vi "CuLab_FM_Demodulate.vi"(8 "error in (no error)":errorcluster, 11 "Signal In":refnum<class "T1D_CSG.lvclass">) -> (0 "error out":errorcluster, 3 "FM Demod Out":refnum<class "T1D_SGL.lvclass">)   [LabVIEW 2020]
uses:
  <vilib>/Ngene/CuLab - GPU Accelerated Toolkit/Toolkit/Low_Level/Tensor_Classes/T_Children/T1D/T1D_Children/T1D_CSG/T1D_CSG.lvclass
  C:/Program Files/National Instruments/LabVIEW 2020/vi.lib/Ngene/CuLab - GPU Accelerated Toolkit/Toolkit/Low_Level/Tensor_Classes/T_Children/T1D/T1D.lvclass
  <vilib>/Ngene/CuLab - GPU Accelerated Toolkit/Toolkit/Low_Level/Tensor_Classes/T_Children/T1D/T1D_Children/T1D_SGL/T1D_SGL.lvclass
  <vilib>/Ngene/CuLab - GPU Accelerated Toolkit/Toolkit/API/Array/Array Subset/T1D/CU_Array_Subset_T1D_CSG.vi
  <vilib>/Ngene/CuLab - GPU Accelerated Toolkit/Toolkit/API/Numeric/Multiply/T1D/CU_Multiply_T1D_CSG.vi
  <vilib>/Ngene/CuLab - GPU Accelerated Toolkit/Toolkit/API/Numeric/Complex  (API)/Complex to Polar/T1D/CU_Complex_to_Polar_T1D_CSG.vi
  <vilib>/Ngene/CuLab - GPU Accelerated Toolkit/Toolkit/API/Numeric/Complex  (API)/Complex Conjugate/T1D/CU_Complex_Conjugate_T1D_CSG.vi
  <vilib>/Ngene/CuLab - GPU Accelerated Toolkit/Toolkit/API/Array/Array Size/CU_Array_Size_T1D.vi
  <vilib>/Ngene/CuLab - GPU Accelerated Toolkit/Toolkit/API/Array/Concat Array/T1D/CU_Concat_Array_T1D_CSG.vi
  <vilib>/Ngene/CuLab - GPU Accelerated Toolkit/Toolkit/Low_Level/Tensor_Classes/T_Children/T1D/T1D_Children/T1D_CSG/Create.vi
  <vilib>/Ngene/CuLab - GPU Accelerated Toolkit/Toolkit/CuLab.lvlib
  C:/Program Files/National Instruments/LabVIEW 2020/vi.lib/Ngene/CuLab - GPU Accelerated Toolkit/Toolkit/Low_Level/Tensor_Classes/Tensor.lvclass
  C:/Program Files/National Instruments/LabVIEW 2020/vi.lib/Ngene/CuLab - GPU Accelerated Toolkit/Toolkit/Low_Level/Tensor_Classes/T_Children/T1D/T1D_Children/T1D_CSG/T1D_CSG.lvclass
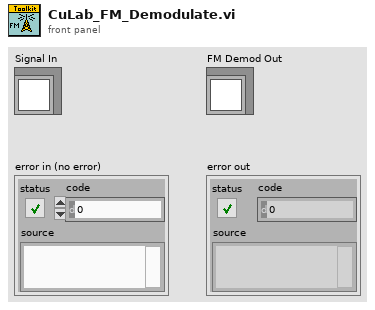
[diagram p1: front panel]
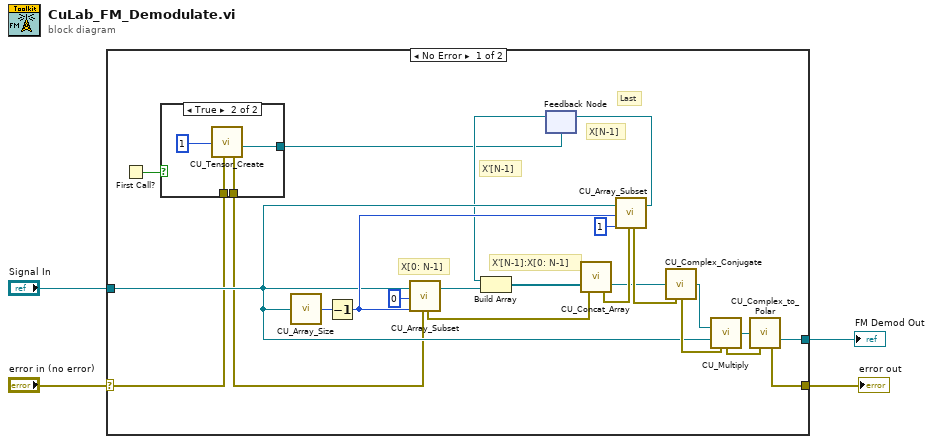
[diagram p0: block diagram]
diagram:
  n1 = case shown="No Error" "error in (no error)" {
    selector: "error in (no error)" -> [w7 w33]
    tunnel: "Signal In" -> [w18 _]
    tunnel: [w5 _] -> w2
    tunnel: [w27 w33] -> w1
    frame No Error {
      # "X'[N-1]:X[0: N-1]"
      # "X'[N-1]"
      # "X[N-1]"
      # "Last"
      # "X[0: N-1]"
      n2 = First Call?() -> (First Call?: T/F=w9:bool)
      n3 = case shown="True" w9 {
        tunnel: [_ w32] -> w8
        tunnel: w7 -> [w28 w30]
        tunnel: [w28 w29] -> w6
        frame False {
        }
        frame True {
          n4 = call-poly <vilib>:"CU_Tensor_Create.vi"("error in (no error)"=w30, "Length"=1) -> ("T1D_CSG out"=w32:refnum<class "T1D_CSG.lvclass">, "error out"=w29:errorcluster)  [unwired: 8 in]
        }
      }
      n5 = call-poly <vilib>:"CU_Array_Size.vi"("Tensor"=w18) -> ("size"=w22:i32)  [unwired: 14 in]
      n6 = Decrement(x=w22) -> (x-1=w20:i32)
      n7 = call-poly <vilib>:"CU_Array_Subset.vi"("Tensor in"=w18, "Index"=0, "Length"=w20, "error in (no error)"=w6) -> ("error out"=w14:errorcluster, "Dest out"=w24:refnum<class "T1D_CSG.lvclass">)  [unwired: 14 in]
      n8 = feedback #1(w8) -> (w15:refnum<class "T1D_CSG.lvclass">)
      n9 = Build Array(w15, w24) -> (w16:refnum<class "T1D_CSG.lvclass">[])
      n10 = call-poly <vilib>:"CU_Concat_Array.vi"("Tensors[]"=w16, "error in (no error)"=w14) -> ("error out"=w12:errorcluster, "Dest out"=w10:refnum<class "T1D_CSG.lvclass">)  [unwired: 16 in]
      n11 = call-poly <vilib>:"CU_Array_Subset.vi"("Tensor in"=w18, "Index"=w20, "Length"=1, "error in (no error)"=w12) -> ("error out"=w11:errorcluster, "Dest out"=w19:refnum<class "T1D_CSG.lvclass">)  [unwired: 14 in]
      n12 = feedback-in #1(w19) -> ()
      n13 = call-poly <vilib>:"CU_Complex_Conjugate.vi"("x"=w10, "error in (no error)"=w11) -> ("Dest out"=w21:refnum<class "T1D_CSG.lvclass">, "error out"=w25:errorcluster)  [unwired: 12 in]
      n14 = call-poly <vilib>:"CU_Multiply.vi"("x"=w21, "y"=w18, "error in (no error)"=w25) -> ("Dest out"=w23:refnum<class "T1D_CSG.lvclass">, "error out"=w26:errorcluster)  [unwired: 11 in]
      n15 = call-poly <vilib>:"CU_Complex_to_Polar.vi"("r * e^(i*theta)"=w23, "error in (no error)"=w26) -> ("theta out"=w5:refnum<class "T1D_SGL.lvclass">, "error out"=w27:errorcluster)  [unwired: 11 in, 1 out]
    }
    frame Error {
    }
  }
  "FM Demod Out" <- w2
  "error out" <- w1
